vi "AO_6711_Load_Wfm.vi"(8 "error in (no error)":errorcluster, 9 "SOFTWARE Inputs":T2={"Application Directory"=path "D:/S.O.F.T.S/LABVIEW/PIL", "Software Version"="1.0.0", "Data Path"=path "D:/PIRENEA/DATA", "XML Path"=path "D:/PIRENEA/DATA", "XML File Filter"="*.xml", "XML Saved Path"=path "D:/PIRENEA/DATA/SAVED", "Excit Scripts Path"=path "D:/PIRENEA/TECHNICAL/EXCIT_SCRIPTS", "Excit Scripts File Filter"="*.txt", "Excit Waveforms Path"=path "D:/PIRENEA/TECHNICAL/EXCIT_WFMS", "Excit Waveforms File Filter"="*.bin", "Timing Scripts Path"=path "D:/PIRENEA/TECHNICAL/TIMING_SCRIPTS", "Timing Scripts File Filter"="*.txt", "Timing Waveforms Path"=path "D:/PIRENEA/TECHNICAL/TIMING_WFMS", "Timing Waveforms File Filter"="*.bin", "Trapping Waveforms Path"=path "D:/PIRENEA/TECHNICAL/TRAPPING_WFMS", "Trapping Waveforms File Filter"="*.bin"}, 10 "TRAPPING Inputs":T1={"Number of Channels"=4, "Init Values"=[2.0, 9.0, 2.0, 9.0], "Opening Values"=[0.0, 0.0, 0.0, 0.0], "Trapping Values"=[2.0, 9.0, 2.0, 9.0], "Emptying Values"=[-10.0, -10.0, -10.0, -10.0], "Adiabatic ON"=FALSE, "Adiabatic Duration"=100, "Adiabatic Waveforms"=["Adiabatic_None_2_2_2000", "Adiabatic_Ramp_9_0_2000", "Adiabatic_None_2_2_2000", "Adiabatic_RC_9_0_2000"], "Ions Refill ON"=FALSE, "Number of Ions Refills"=1, "Trapping Delay"=400.0, "Trapping Duration"=300.0} {"Trapping Duration" min=2.0; "Trapping Delay" min=2.0; "Number of Ions Refills" min=1 max=1000; "Trapping Values" min=-10.0 max=10.0; "Init Values" min=-10.0 max=10.0; "Emptying Values" min=-10.0 max=10.0; "Opening Values" min=-10.0 max=10.0}, 11 "Instrument handle in":refnum<k21> caption="tâche/voies en entrée") -> (0 "error out":errorcluster, 1 "number of samples written per channel":u32 caption="nombre d'échantillons écrits par voie", 2 "number of samples":i32, 3 "Instrument handle out":refnum<k21>)   [LabVIEW 2018]
doc: "This VI demonstrates how to load dynamic waveforms into the board.\n\n1. The waveform binary files are read one by one from the waveform folder.\n2. The data are converted to U32 format and loaded into the on-board memory.\n\nThis VI returns the max memory size of the board, the memory used after loading, and a list of the waveforms loaded. No check of memory overflow is done."
uses:
  controls/SOFTWARE_Inputs.ctl
  controls/TRAPPING_Inputs.ctl
  <vilib>/DAQmx/write.llb/DAQmx Write (Analog 2D DBL NChan NSamp).vi
  <vilib>/DAQmx/miscellaneous.llb/DAQmx Fill In Error Info.vi
  <resource>/objmgr/daqmx.rc
panel:
  # "GO_out"
  # "Gout"
  # "GI_in"
  # "Gin"
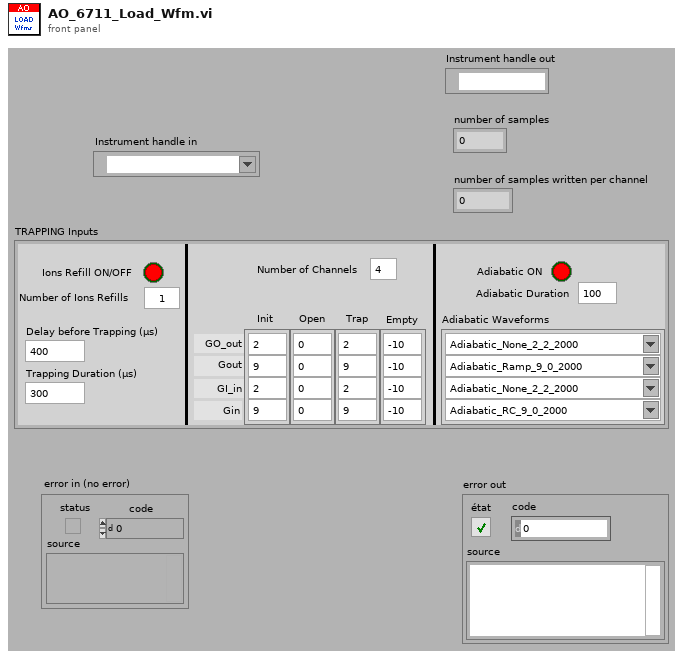
[diagram p1: front panel]
types:
  T1 = typedef "TRAPPING_Inputs.ctl" = cluster{"Number of Channels":i32, "Init Values":dbl[], "Opening Values":dbl[], "Trapping Values":dbl[], "Emptying Values":dbl[], "Adiabatic ON":bool, "Adiabatic Duration":i32, "Adiabatic Waveforms":string[], "Ions Refill ON":bool, "Number of Ions Refills":i32, "Trapping Delay":dbl, "Trapping Duration":dbl}
  T2 = typedef "SOFTWARE_Inputs.ctl" = cluster{"Application Directory":path, "Software Version":string, "Data Path":path, "XML Path":path, "XML File Filter":string, "XML Saved Path":path, "Excit Scripts Path":path, "Excit Scripts File Filter":string, "Excit Waveforms Path":path, "Excit Waveforms File Filter":string, "Timing Scripts Path":path, "Timing Scripts File Filter":string, "Timing Waveforms Path":path, "Timing Waveforms File Filter":string, "Trapping Waveforms Path":path, "Trapping Waveforms File Filter":string}
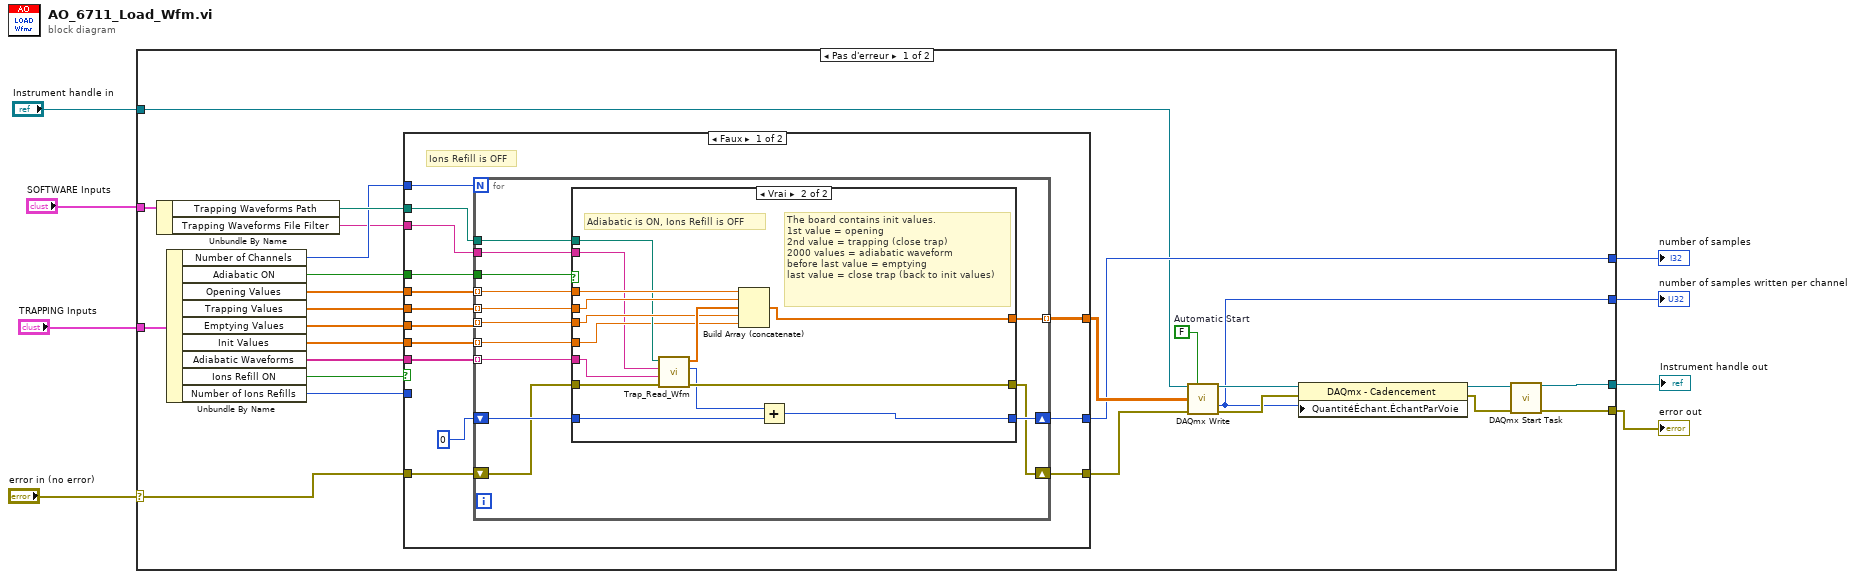
[diagram p0: block diagram]
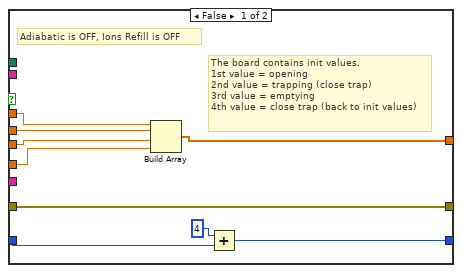
[diagram p2: hidden frame]
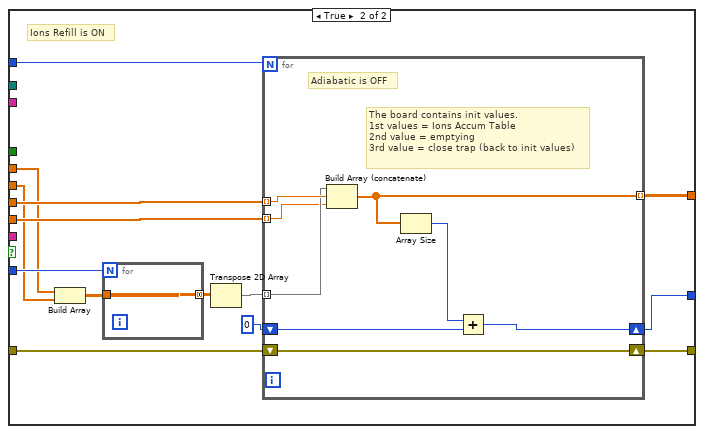
[diagram p3: hidden frame]
diagram:
  n1 = case shown="Pas d'erreur" "error in (no error)" {
    selector: "error in (no error)" -> [w18 w109]
    tunnel: [w23 w109] -> w8
    tunnel: "SOFTWARE Inputs" -> [w34 _]
    tunnel: [w22 _] -> w7
    tunnel: [w12 _] -> w6
    tunnel: "Instrument handle in" -> [w21 w108]
    tunnel: [w17 w108] -> w3
    tunnel: "TRAPPING Inputs" -> [w9 _]
    frame No Error {
      w33 = FALSE  # Automatic Start
      n2 = Unbundle By Name(w34) -> ("Trapping Waveforms Path"=w31:path, "Trapping Waveforms File Filter"=w20:string)
      n3 = Unbundle By Name(w9) -> ("Number of Channels"=w30:i32, "Adiabatic ON"=w25:bool, "Opening Values"=w27:dbl[], "Trapping Values"=w26:dbl[], "Emptying Values"=w29:dbl[], "Init Values"=w24:dbl[], "Adiabatic Waveforms"=w28:string[], "Ions Refill ON"=w11:bool, "Number of Ions Refills"=w10:i32)
      n4 = case shown="Faux" w11 {
        tunnel: [w48 w87] -> w32
        tunnel: w31 -> [w46 _]
        tunnel: w30 -> [w45 w95]
        tunnel: w29 -> [w44 w94]
        tunnel: w28 -> [w43 _]
        tunnel: w27 -> [w42 w86]
        tunnel: w26 -> [w41 w85]
        tunnel: w25 -> [w40 _]
        tunnel: w24 -> [w39 w93]
        tunnel: [w38 w88] -> w22
        tunnel: w20 -> [w37 _]
        tunnel: [w36 w90] -> w19
        tunnel: w18 -> [w35 w91]
        tunnel: w10 -> [_ w96]
        frame False {
          # "Ions Refill is OFF"
          n5 = for {
            N: w45 -> [_]
            tunnel: w40 -> [w57]
            tunnel: w42 -> [w60] mode=indexing
            tunnel: w44 -> [w59] mode=indexing
            tunnel: w43 -> [w56] mode=indexing
            tunnel: w41 -> [w58] mode=indexing
            tunnel: [w61] -> w48 mode=indexing
            tunnel: w46 -> [w55]
            shift-right: [w53] -> w38
            shift-left: 0 -> [w54]
            tunnel: w39 -> [w52] mode=indexing
            tunnel: w37 -> [w51]
            shift-right: [w50] -> w36
            shift-left: w35 -> [w49]
            n6 = case shown="Vrai" w57 {
              tunnel: [w63 w79] -> w61
              tunnel: w60 -> [w67 w83]
              tunnel: w59 -> [w65 w81]
              tunnel: w58 -> [w66 w80]
              tunnel: w56 -> [_ w84]
              tunnel: w55 -> [_ w78]
              tunnel: w54 -> [w70 w77]
              tunnel: [w68 w76] -> w53
              tunnel: w52 -> [w64 w75]
              tunnel: w51 -> [_ w74]
              tunnel: [w62 w73] -> w50
              tunnel: w49 -> [w62 w72]
              frame False {
                # "Adiabatic is OFF, Ions Refill is OFF"
                # "The board contains init values.\n1st value = opening\n2nd value = trapping (close trap)\n3rd value = emptying\n4th value = close trap (back to init values)"
                n7 = Build Array(w67, w66, w65, w64) -> (w63:dbl[])
                n8 = Add(x=4, y=w70) -> (x+y=w68:i32)
              }
              frame True {
                # "Adiabatic is ON, Ions Refill is OFF"
                # "The board contains init values.\n1st value = opening\n2nd value = trapping (close trap)\n2000 values = adiabatic waveform\nbefore last value = emptying\nlast value = close trap (back to init values)"
                n9 = call "Trap_Read_Wfm.vi"("error in (no error)"=w72, "Waveform Name"=w84, "Trapping Waveforms File Filter"=w74, "Trapping Waveforms Path"=w78) -> ("error out"=w73:errorcluster, "Wfm size"=w71:i32, "Wfm data"=w82:dbl[])  [unwired: 5 in]
                n10 = Build Array (concatenate)(w83, w80, w82, w81, w75) -> (w79:dbl[])
                n11 = Add(x=w71, y=w77) -> (x+y=w76:i32)
              }
            }
          }
        }
        frame True {
          # "Ions Refill is ON"
          n12 = Build Array(w86, w85) -> (w98:dbl[][])
          n13 = for {
            N: w96 -> [_]
            tunnel: w98 -> [w107]
            tunnel: [w107] -> w97 mode=concatenating
          }
          n14 = Transpose 2D Array(2D array=w97) -> (transposed array=w92:dbl[][])
          n15 = for {
            N: w95 -> [_]
            tunnel: w94 -> [w106] mode=indexing
            tunnel: w92 -> [w105] mode=indexing
            tunnel: [w100] -> w87 mode=indexing
            shift-right: [w103] -> w88
            shift-left: 0 -> [w104]
            tunnel: w93 -> [w102] mode=indexing
            shift-right: [w101] -> w90
            shift-left: w91 -> [w101]
            # "Adiabatic is OFF"
            # "The board contains init values.\n1st values = Ions Accum Table\n2nd value = emptying\n3rd value = close trap (back to init values)"
            n16 = Build Array (concatenate)(w105, w106, w102) -> (w100:dbl[])
            n17 = Array Size(array=w100) -> (size(s)=w99:i32)
            n18 = Add(x=w99, y=w104) -> (x+y=w103:i32)
          }
        }
      }
      n19 = call-poly <vilib>:"DAQmx Write.vi"("task/channels in"=w21, "auto start"=w33, "data"=w32, "error in"=w19) -> ("task out"=w16:refnum<k21>, "number of samples written per channel"=w12:u32, "error out"=w14:errorcluster)  [unwired: 9 in]
      n20 = property class="DAQmx - Cadencement"(reference=w16, error in=w14, "QuantitéÉchant.ÉchantParVoie"=w12) -> (reference out=w15:refnum<k21>, error out=w13:errorcluster)
      n21 = call <vilib>:"DAQmx Start Task.vi"("task/channels in"=w15, "error in"=w13) -> ("task out"=w17:refnum<k21>, "error out"=w23:errorcluster)  [unwired: 12 in]
    }
    frame Error {
    }
  }
  "error out" <- w8
  "number of samples" <- w7
  "number of samples written per channel" <- w6
  "Instrument handle out" <- w3
